vi "Command Decoder.vi"(1 "Command Mode":enum16{"Write", "Read"}(ring), 2 "Command Type":T1(ring)) -> (0 "Start symbol":string)   [LabVIEW 2017, in "Roboteq Controller KBL1xxx.lvlib"]
uses:
  <instrlib>/Roboteq Controller KBL1xxx/Roboteq Controller KBL1xxx.lvlib
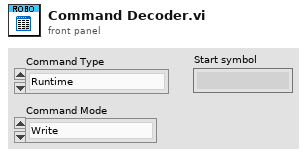
[diagram p1: front panel]
types:
  T1 = enum16{"Runtime", "Configuration", "Maintenance"}
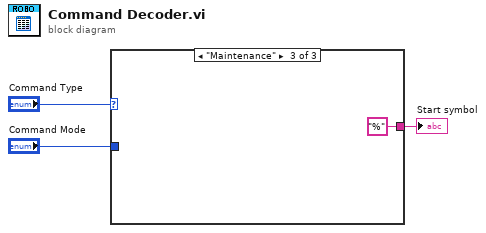
[diagram p0: block diagram]
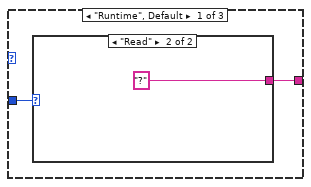
[diagram p2: hidden frame]
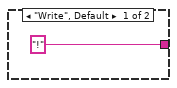
[diagram p3: hidden frame]
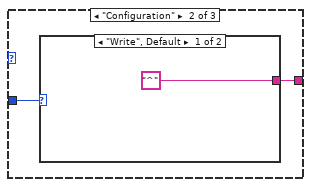
[diagram p4: hidden frame]
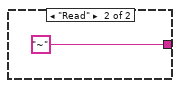
[diagram p5: hidden frame]
diagram:
  n1 = case shown="\"Maintenance\"" "Command Type" {
    tunnel: "Command Mode" -> [w5 w9 _]
    tunnel: [w4 w8 "%"] -> w1
    frame "Runtime", Default {
      n2 = case shown="\"Read\"" w5 {
        tunnel: ["!" "?"] -> w4
        frame "Write", Default {
        }
        frame "Read" {
        }
      }
    }
    frame "Configuration" {
      n3 = case shown="\"Write\", Default" w9 {
        tunnel: ["^" "~"] -> w8
        frame "Write", Default {
        }
        frame "Read" {
        }
      }
    }
    frame "Maintenance" {
    }
  }
  "Start symbol" <- w1
